vi "Initialize.vi"(8 "error in":errorcluster, 11 "Plugin in":refnum<class "RPM Measurement.lvclass">) -> (0 "error out":errorcluster, 3 "Plugin out":refnum<class "RPM Measurement.lvclass">)   [LabVIEW 2020, in "RPM Measurement.lvlib" / "RPM Measurement.lvclass"]
uses:
  RPM Measurement.lvclass
  C:/Program Files/National Instruments/LabVIEW 2020/vi.lib/FlexLogger/SDK/PluginSDK.lvlibp/PEFClasses/SDK/Plugin/Plugin.lvclass
  <vilib>/FlexLogger/SDK/PluginSDK.lvlibp/PEFClasses/SDK/System Interface/Resampling Mode.ctl
  <vilib>/FlexLogger/SDK/PluginSDK.lvlibp/PEFClasses/SDK/Processing Element/Timing Parameters.ctl
  <vilib>/FlexLogger/SDK/PluginSDK.lvlibp/PEFClasses/SDK/Processing Element/Timing Method.ctl
  <vilib>/FlexLogger/SDK/PluginSDK.lvlibp/PEFClasses/SDK/Producer Channel/Producer Channel.lvclass
  C:/Program Files/National Instruments/LabVIEW 2020/vi.lib/FlexLogger/SDK/PluginSDK.lvlibp/PEFClasses/SDK/Channel/Channel.lvclass
  <vilib>/FlexLogger/SDK/PluginSDK.lvlibp/PEFClasses/SDK/Plugin/ParameterAccess/Write Single Channel.vi
  <vilib>/FlexLogger/SDK/PluginSDK.lvlibp/PEFClasses/SDK/Plugin/ParameterAccess/Write DBL.vi
  <vilib>/FlexLogger/SDK/PluginSDK.lvlibp/PEFClasses/SDK/Producer Channel/Create Producer Channel.vi
  <vilib>/FlexLogger/SDK/PluginSDK.lvlibp/PEFClasses/SDK/Plugin/Plugin.lvclass
  <vilib>/FlexLogger/SDK/PluginSDK.lvlibp
  <vilib>/FlexLogger/SDK/PluginSDK.lvlibp/PEFClasses/SDK/System Interface/System Interface.lvclass
  C:/Program Files/National Instruments/LabVIEW 2020/vi.lib/FlexLogger/SDK/PluginSDK.lvlibp/PEFClasses/SDK/Processing Element/Processing Element.lvclass
  C:/Users/NIIndiaAE/Desktop/FlexLogger Plugin/RPM Plugin/RPM Measurement.lvclass
  <vilib>/FlexLogger/SDK/PluginSDK.lvlibp/PEFClasses/SDK/Processing Element/Processing Element.lvclass
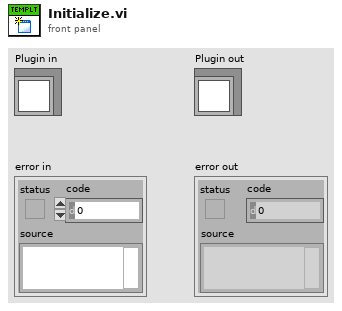
[diagram p1: front panel]
types:
  T1 = typedef "PluginSDK.lvlibp/Processing Element.lvclass/Timing Parameters.ctl" = cluster{"Timing Method":T2, "Timing Period (ms)":i32}
  T2 = typedef "PluginSDK.lvlibp/Processing Element.lvclass/Timing Method.ctl" = enum16{"Periodic", "Immediate", "On Data Ready", "Triggered"}
  T3 = typedef "PluginSDK.lvlibp/System Interface.lvclass/Resampling Mode.ctl" = enum16{"No Resampling", "Custom Rate", "Maximum Rate", "Minimum Rate"}
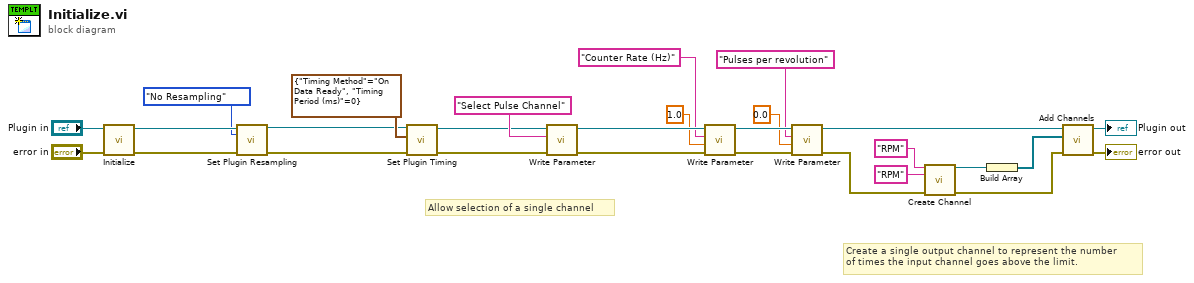
[diagram p0: block diagram]
diagram:
  # "Create a single output channel to represent the number \nof times the input channel goes above the limit."
  # "Allow selection of a single channel"
  n1 = call-parent "Initialize.vi"("error in (no error)"="error in", "Plugin in"="Plugin in") -> ("error out"=w23:errorcluster, "Plugin out"=w24:refnum<class "RPM Measurement.lvclass">)  [unwired: 8 in]
  n2 = call <vilib>:"Set Plugin Resampling.vi"("Plugin in"=w24, "Resampling Mode"=Resampling_Mode."No Resampling", "error in (no error)"=w23) -> ("Plugin out"=w12:refnum<class "RPM Measurement.lvclass">, "error out"=w11:errorcluster)  [unwired: 11 in]
  n3 = call <vilib>:"Set Plugin Timing.vi"("error in (no error)"=w11, "Timing Parameters"=T1 {"Timing Method"=enum."On Data Ready", "Timing Period (ms)"=0}, "Plugin in"=w12) -> ("error out"=w10:errorcluster, "Plugin out"=w9:refnum<class "RPM Measurement.lvclass">)  [unwired: 7 in]
  n4 = call-poly <vilib>:"Write Parameter.vi"("error in (no error)"=w10, "Name (Unique Channel Identifier)"="Select Pulse Channel" ("Name"), "Plugin in"=w9) -> ("error out"=w16:errorcluster, "Plugin out"=w17:refnum<class "RPM Measurement.lvclass">)  [unwired: 7 in]
  n5 = call-poly <vilib>:"Write Parameter.vi"("error in (no error)"=w16, "Value"=1.0, "Name"="Counter Rate (Hz)", "Plugin in"=w17) -> ("error out"=w4:errorcluster, "Plugin out"=w6:refnum<class "RPM Measurement.lvclass">)  [unwired: 6 in]
  n6 = call-poly <vilib>:"Write Parameter.vi"("error in (no error)"=w4, "Value"=0.0, "Name"="Pulses per revolution", "Plugin in"=w6) -> ("error out"=w3:errorcluster, "Plugin out"=w5:refnum<class "RPM Measurement.lvclass">)  [unwired: 6 in]
  n7 = call-poly <vilib>:"Create Channel.vi"("Unique Channel Identifier"="RPM", "Default Channel Name"="RPM" ("Unique Channel Identifier"), "error in (no error)"=w3) -> ("Producer Channel"=w22:refnum<class "Producer Channel.lvclass">, "error out"=w20:errorcluster)  [unwired: 11 in]
  n8 = Build Array(w22) -> (w21:refnum<class "Producer Channel.lvclass">[])
  n9 = call <vilib>:"Add Channels.vi"("error in (no error)"=w20, "Channels"=w21, "Plugin in"=w5) -> ("error out"=→"error out":errorcluster, "Plugin out"=→"Plugin out":refnum<class "RPM Measurement.lvclass">)  [unwired: 7 in]
